vi "CreateDataFlowMapsBurstMode.vi"(8 "error in (no error)":errorcluster, 11 "923x Acquisition Config":T1 {"HighPassFilterState"."Filter State" format="%.2f"; "HighPassFilterState"."IIR Filter Cluster"."Forward Coefficients" format="%.2f"; "HighPassFilterState"."IIR Filter Cluster"."Reverse Coefficients" format="%.2f"; "FixedSizeX32"."InputConfig" items=["AC Coupled", "DC Coupled", "IEPE AC Coupled"]}) -> (0 "error out":errorcluster, 1 "maps":T10[](array[typedef]), 3 "923x Acquisition Config out":T1 {"HighPassFilterState"."Filter State" format="%.2f"; "HighPassFilterState"."IIR Filter Cluster"."Forward Coefficients" format="%.2f"; "HighPassFilterState"."IIR Filter Cluster"."Reverse Coefficients" format="%.2f"; "FixedSizeX32"."InputConfig" items=["AC Coupled", "DC Coupled", "IEPE AC Coupled"]})   [LabVIEW 2017, in "CmsAcquisition.lvlib"]
uses:
  <vilib>/addons/InsightCM/Devices/Shared/Cms/CmsAcquisition/CmsAcquisition.lvlib
  <vilib>/addons/InsightCM/Devices/Shared/Cms/CmsAcquisition/controls/Configuration.ctl
  <vilib>/addons/InsightCM/Devices/Shared/Cms/CmsAcquisition/controls/TachometerConfig.ctl
  <vilib>/addons/InsightCM/Devices/Shared/Cms/CmsAcquisition/controls/FixedSizeArrays.ctl
  <vilib>/LabVIEW Targets/FPGA/cRIO/shared/nicrio_ModuleControls/nicrio_cRIO-9232_ConfigModeRing.ctl
  <vilib>/addons/InsightCM/Devices/Shared/Cms/cRIOWfmAcq/subVIs/RIO Wfm Cust Ctrls/rwfm_SamplingInfo.ctl
  <vilib>/addons/InsightCM/Devices/Shared/Cms/CmsAcquisition/controls/Group.ctl
  <vilib>/addons/InsightCM/Devices/Shared/Cms/CmsAcquisition/controls/Channel.ctl
  <vilib>/addons/InsightCM/Utilities/Analysis/Vibration/controls/HighPassFilterState.ctl
  <vilib>/addons/InsightCM/Devices/Shared/Cms/CmsAcquisition/controls/BurstMode.ctl
  <vilib>/addons/PointValueMap/controls/PointMap.ctl
  <vilib>/addons/PointValueMap/subVIs/Point_Write_double.vi
  <vilib>/addons/PointValueMap/subVIs/Point_Write_i32.vi
  <vilib>/addons/PointValueMap/subVIs/Point_Write_string.vi
  <vilib>/addons/PointValueMap/PointValueMap.lvlib
  <vilib>/addons/InsightCM/Devices/Shared/Cms/cRIOWfmAcq/cRIOWfmLib.lvlib
  <vilib>/addons/InsightCM/Utilities/Analysis/Vibration/VibrationAnalysisFunctions.lvlib
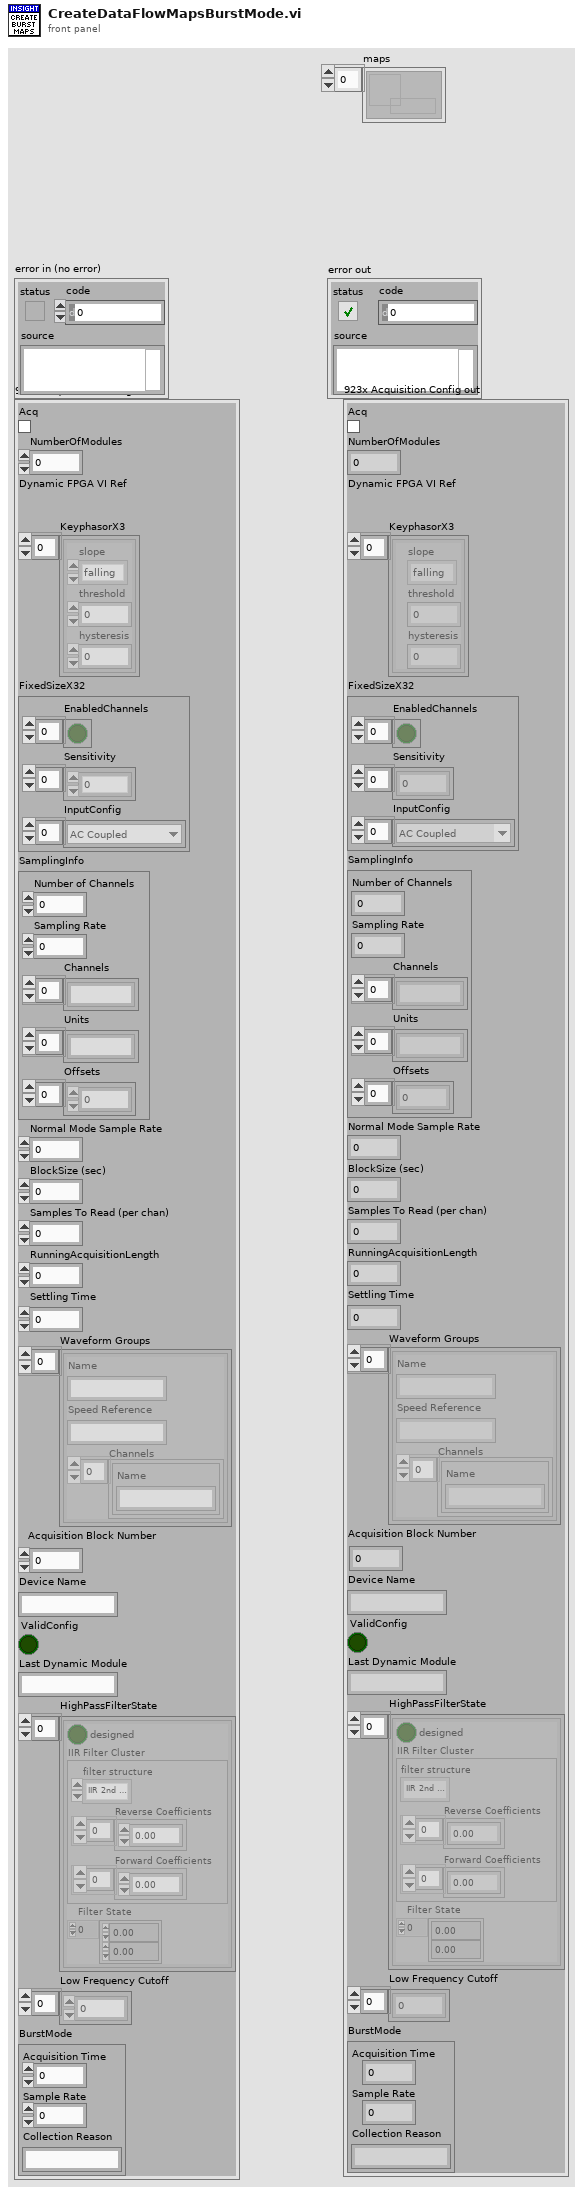
[diagram p1: front panel]
types:
  T1 = typedef "CmsAcquisition.lvlib/Configuration.ctl" = cluster{"Acq":bool, "NumberOfModules":i16, "Dynamic FPGA VI Ref":refnum<k20>, "KeyphasorX3":T2[], "FixedSizeX32":T3, "SamplingInfo":T5, "Normal Mode Sample Rate":dbl, "BlockSize (sec)":dbl, "Samples To Read (per chan)":i32, "RunningAcquisitionLength":dbl, "Settling Time":dbl, "Waveform Groups":T6[], "Acquisition Block Number":i32, "Device Name":string, "ValidConfig":bool, "Last Dynamic Module":string, "HighPassFilterState":T8[], "Low Frequency Cutoff":dbl[], "BurstMode":T9}
  T2 = typedef "CmsAcquisition.lvlib/TachometerConfig.ctl" = cluster{"slope":enum16{"falling", "rising"}, "threshold":dbl, "hysteresis":dbl}
  T3 = typedef "CmsAcquisition.lvlib/FixedSizeArrays.ctl" = cluster{"EnabledChannels":bool[], "Sensitivity":dbl[], "InputConfig":T4[]}
  T4 = typedef "nicrio_cRIO-9232_ConfigModeRing.ctl" = u8
  T5 = typedef "cRIOWfmLib.lvlib/rwfm_SamplingInfo.ctl" = cluster{"Number of Channels":i32, "Sampling Rate":dbl, "Channels":string[], "Units":string[], "Offsets":sgl[]}
  T6 = typedef "CmsAcquisition.lvlib/Group.ctl" = cluster{"Name":string, "Speed Reference":string, "Channels":T7[]}
  T7 = typedef "CmsAcquisition.lvlib/Channel.ctl" = cluster{"Name":string}
  T8 = typedef "VibrationAnalysisFunctions.lvlib/HighPassFilterState.ctl" = cluster{"designed":bool, "IIR Filter Cluster":cluster{"filter structure":enum32{"IIR 2nd Order", "IIR 4th Order"}, "Reverse Coefficients":dbl[], "Forward Coefficients":dbl[]}, "Filter State":dbl[]}
  T9 = typedef "CmsAcquisition.lvlib/BurstMode.ctl" = cluster{"Acquisition Time":dbl, "Sample Rate":dbl, "Collection Reason":string}
  T10 = typedef "PointValueMap.lvlib/PointMap.ctl" = refnum<data-value>
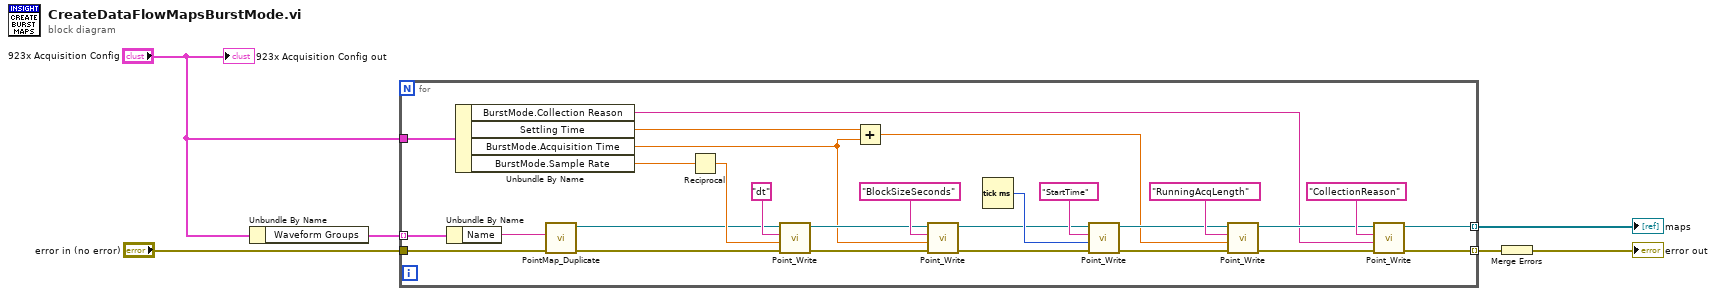
[diagram p0: block diagram]
diagram:
  n1 = Unbundle By Name("923x Acquisition Config") -> ("Waveform Groups"=w2:T6[])
  n2 = for {
    tunnel: w2 -> [w34] mode=indexing
    tunnel: "error in (no error)" -> [w32]
    tunnel: "923x Acquisition Config" -> [w26]
    tunnel: [w9] -> w1 mode=indexing
    tunnel: [w8] -> w3 mode=indexing
    n3 = Unbundle By Name(w34) -> ("Name"=w33:string)
    n4 = Unbundle By Name(w26) -> ("BurstMode.Collection Reason"=w7:string, "Settling Time"=w14:dbl, "BurstMode.Acquisition Time"=w15:dbl, "BurstMode.Sample Rate"=w21:dbl)
    n5 = call <vilib>:"PointMap_Duplicate.vi"("error in (no error)"=w32, "Source Map Name"=w33) -> ("error out"=w24:errorcluster, "Map Out"=w25:T10)  [unwired: 8 in]
    n6 = Reciprocal(x=w21) -> (1/x=w27:dbl)
    n7 = call-poly <vilib>:"Point_Write.vi"("Error In"=w24, "Value"=w27, "Tag"="dt", "Map"=w25) -> ("Error Out"=w29:errorcluster, "Map Out"=w28:T10)  [unwired: 6 in]
    n8 = Add(x=w14, y=w15) -> (x+y=w13:dbl)
    n9 = call-poly <vilib>:"Point_Write.vi"("Error In"=w29, "Value"=w15, "Tag"="BlockSizeSeconds", "Map"=w28) -> ("Error Out"=w19:errorcluster, "Map Out"=w20:T10)  [unwired: 6 in]
    n10 = Tick Count (ms)() -> (millisecond timer value=w22:u32)
    n11 = call-poly <vilib>:"Point_Write.vi"("Error In"=w19, "Value"=w22, "Tag"="StartTime", "Map"=w20) -> ("Error Out"=w16:errorcluster, "Map Out"=w17:T10)  [unwired: 6 in]
    n12 = call-poly <vilib>:"Point_Write.vi"("Error In"=w16, "Value"=w13, "Tag"="RunningAcqLength", "Map"=w17) -> ("Error Out"=w10:errorcluster, "Map Out"=w11:T10)  [unwired: 6 in]
    n13 = call-poly <vilib>:"Point_Write.vi"("Error In"=w10, "Value"=w7, "Tag"="CollectionReason", "Map"=w11) -> ("Error Out"=w9:errorcluster, "Map Out"=w8:T10)  [unwired: 6 in]
  }
  "maps" <- w3
  n14 = Merge Errors(w1) -> (→"error out":errorcluster)
  "923x Acquisition Config out" <- "923x Acquisition Config"
